vi "Convert Error Cluster to Table.vi"(11 "Error Codes":cluster{i32, string}[](array[cluster])) -> (2 "Code":i32[](array[numeric]), 3 "String":string[](array[string]))   [LabVIEW 2019, in "Ghost Bus Addon System Explorer.lvlib"] (continued)
of the remote endpoint does not match the data type of the local endpoint. The data types of the endpoints must match."}, {-314240, "LabVIEW: (Hex 0xFFFB3480) The stream detected an unrecoverable loss of data.  Contact National Instruments for support."}, {-314235, "LabVIEW: (Hex 0xFFFB3485) The remote endpoint was restarted because the computer that hosts the endpoint crashed, was rebooted, or experienced a hang."}, {-314230, "LabVIEW: (Hex 0xFFFB348A) LabVIEW could not create the local endpoint because the computer that hosts the endpoint ran out of memory."}, {-314227, "LabVIEW: (Hex 0xFFFB348D) The URL you specified with the reader url or writer url terminal does not include the name of the remote endpoint. You must specify a valid endpoint URL in one of these terminals to connect two endpoints together."}, {-314226, "LabVIEW: (Hex 0xFFFB348E) Incompatible format."}, {-314220, "LabVIEW: (Hex 0xFFFB3494) The remote endpoint has been destroyed."}, {-314215, "LabVIEW: (Hex 0xFFFB3499) You cannot read or write a number of elements that is larger than the size of the endpoint buffer."}, {-314202, "LabVIEW: (Hex 0xFFFB34A6) You cannot flush a network stream from the reader endpoint. Call the Flush Stream function from the writer endpoint only."}, {-314201, "LabVIEW: (Hex 0xFFFB34A7) The local endpoint lost connection and reconnected with the remote endpoint, but some data was lost."}, {-314109, "LabVIEW: (Hex 0xFFFB3503) The name of one endpoint cannot be the partial name of another endpoint within the same application.  Change the name of this endpoint so that it does not overlap with an existing name, or destroy the other endpoint before creating this endpoint."}, {-314108, "LabVIEW: (Hex 0xFFFB3504) The name of one endpoint cannot be the partial name of another endpoint within the same application.  Change the name of this endpoint so that it does not overlap with an existing name, or destroy the other endpoint before creating this endpoint."}, {-314107, "LabVIEW: (Hex 0xFFFB3505) The local endpoint is already connected to another endpoint. Each endpoint can connect to only one other endpoint at a time."}, {-314106, "LabVIEW: (Hex 0xFFFB3506) The local endpoint is not connected to a remote endpoint. Specify the URL of a remote endpoint in the writer url terminal of the Create Network Stream Reader Endpoint function or the reader url terminal of the Create Network Stream Writer Endpoint function to prompt a connection between two endpoints."}, {-314105, "LabVIEW: (Hex 0xFFFB3507) You can call the Write Single Element to Stream and Write Multiple Elements to Stream functions from the writer endpoint only."}, {-314104, "LabVIEW: (Hex 0xFFFB3508) You can call the Read Single Element from Stream and Read Multiple Elements from Stream functions from the reader endpoint only."}, {-314103, "LabVIEW: (Hex 0xFFFB3509) You did not specify an endpoint name. Specify a valid name or endpoint URL with the reader name terminal of the Create Network Stream Reader Endpoint function or the writer name terminal of the Create Network Stream Writer Endpoint function."}, {-314102, "LabVIEW: (Hex 0xFFFB350A) The buffer size of the endpoint must be greater than zero elements."}, {-314101, "LabVIEW: (Hex 0xFFFB350B) An endpoint with the same name already exists."}, {-314100, "LabVIEW: (Hex 0xFFFB350C) The specified endpoint does not exist."}, {-314054, "LabVIEW: (Hex 0xFFFB353A) The Network Streams Engine cannot be uninitialized."}, {-314053, "LabVIEW: (Hex 0xFFFB353B) The Network Streams Engine failed to initialize."}, {-314052, "LabVIEW: (Hex 0xFFFB353C) The Network Streams Engine is not initialized."}, {-314051, "LabVIEW: (Hex 0xFFFB353D) The Network Streams Engine was already initialized."}, {-314050, "LabVIEW: (Hex 0xFFFB353E) The Network Streams Engine does not exist."}, {-314009, "LabVIEW: (Hex 0xFFFB3567) The value wired to the Wait Condition input is invalid. Refer to the LabVIEW Help for valid values."}, {-314008, "LabVIEW: (Hex 0xFFFB3568) The value wired to the Element Allocation Mode input is invalid. Refer to the LabVIEW Help for valid values."}, {-314007, "LabVIEW: (Hex 0xFFFB3569) You cannot read multiple array elements of different dimensions. You can read multiple array elements of the same dimension only."}, {-314006, "LabVIEW: (Hex 0xFFFB356A) You cannot specify a relative URL with the reader url and writer url terminals. You must use an absolute URL instead. For example,  if you are connecting to an endpoint with the name Endpoint1 on a computer with the IP address 10.0.0.62, use the URL //10.0.0.62/stream1."}, {-314005, "LabVIEW: (Hex 0xFFFB356B) The ni_nwstreams library contains invalid parameters."}, {-314004, "LabVIEW: (Hex 0xFFFB356C) LabVIEW could not create the endpoint within the timeout period. Ensure that you specify the URL of a remote endpoint with the reader url terminal of the Create Network Stream Writer Endpoint function or the writer url terminal of the Create Network Stream Reader Endpoint function."}, {-314003, "LabVIEW: (Hex 0xFFFB356D) LabVIEW could not create a network stream. You must specify the URL of a remote endpoint with either the reader url terminal of the Create Network Stream Writer Endpoint function or the writer url terminal of the Create Network Stream Reader Endpoint function."}, {-314002, "LabVIEW: (Hex 0xFFFB356E) You cannot call this property from the reader endpoint. You can call this property from the writer endpoint only."}, {-314001, "LabVIEW: (Hex 0xFFFB356F) You cannot call this property from the writer endpoint. You can call this property from the reader endpoint only."}, {-314000, "LabVIEW: (Hex 0xFFFB3570) LabVIEW cannot load the ni_nwstreams library. If you are using a desktop computer, you might need to repair your LabVIEW installation or reinstall LabVIEW or the LabVIEW Run-Time Engine. If you are using an RT target, verify that you installed the network streams feature with Measurement and Automation Explorer (MAX)."}, {-311119, "LabVIEW: (Hex 0xFFFB40B1) Failed to connect to the MAX database (MXS) when undeploying the EPICS Client I/O server."}, {-311118, "LabVIEW: (Hex 0xFFFB40B2) Failed to connect to the MAX database (MXS) when deploying the EPICS Client I/O server."}, {-311117, "LabVIEW: (Hex 0xFFFB40B3) Failed to connect to the MAX database (MXS) when creating the EPICS Client I/O server."}, {-311116, "LabVIEW: (Hex 0xFFFB40B4) The specified access type is invalid for the EPICS Client I/O server."}, {-311115, "LabVIEW: (Hex 0xFFFB40B5) The specified data type is invalid for the EPICS Client I/O server."}, {-311114, "LabVIEW: (Hex 0xFFFB40B6) Unable to find the specified field name on the EPICS Client I/O server."}, {-311113, "LabVIEW: (Hex 0xFFFB40B7) Unable to find the specified record name on the EPICS Client I/O server."}, {-311111, "LabVIEW: (Hex 0xFFFB40B9) Failed to locate a network interface. Make sure you have properly configured a network interface. Then deploy the EPICS Server I/O server again."}, {-311110, "LabVIEW: (Hex 0xFFFB40BA) Failed to load EPICS Base libraries. Make sure you have properly installed EPICS Base libraries."}, {-311109, "LabVIEW: (Hex 0xFFFB40BB) The specified process variable (PV) name includes an invalid character. The valid character set for a PV name is: a-z, A-Z, 0-9, _, -, :, ., [, ], <, >, ;."}, {-311108, "LabVIEW: (Hex 0xFFFB40BC) Unable to locate the process variable (PV)."}, {-311107, "LabVIEW: (Hex 0xFFFB40BD) Failed to connect to the MAX database (MXS) when removing an empty process or folder."}, {-311106, "LabVIEW: (Hex 0xFFFB40BE) Failed to connect to the MAX database (MXS) when undeploying the EPICS Server I/O server."}, {-311105, "LabVIEW: (Hex 0xFFFB40BF) Failed to connect to the MAX database (MXS) when deploying the EPICS Server I/O server."}, {-311104, "LabVIEW: (Hex 0xFFFB40C0) Failed to connect to the MAX database (MXS) when creating a process or folder."}, {-311103, "LabVIEW: (Hex 0xFFFB40C1) Failed to connect to the MAX database (MXS) when creating the EPICS Server I/O server."}, {-311102, "LabVIEW: (Hex 0xFFFB40C2) The specified process variable (PV) name conflicts with an existing PV name."}, {-311101, "LabVIEW: (Hex 0xFFFB40C3) The variable path must be a valid absolute URL or a machine-relative URL."}, {-311100, "LabVIEW: (Hex 0xFFFB40C4) Not a URL or an invalid URL. The EPICS Client URL or EPICS Server URL must be an absolute URL or a machine-relative URL."}, {-311071, "LabVIEW: (Hex 0xFFFB40E1) Unable to run the built application on the target. A user must log into a Windows session on the target."}, {-311070, "LabVIEW: (Hex 0xFFFB40E2) Unable to run the built application on the target. The target returns an unexpected error."}, {-311052, "LabVIEW: (Hex 0xFFFB40F4) Cannot commit all files."}, {-311051, "LabVIEW: (Hex 0xFFFB40F5) FBWF returned an unknown error."}, {-311050, "LabVIEW: (Hex 0xFFFB40F6) Cannot find the FBWF cache entry."}, {-311049, "LabVIEW: (Hex 0xFFFB40F7) The system does not have enough memory to list all the FBWF cache entries."}, {-311048, "LabVIEW: (Hex 0xFFFB40F8) The file path to remove does not exist in the exclusion list for the next session."}, {-311047, "LabVIEW: (Hex 0xFFFB40F9) The file to restore does not exist in the FBWF cache."}, {-311046, "LabVIEW: (Hex 0xFFFB40FA) Cannot restore a read-only file."}, {-311045, "LabVIEW: (Hex 0xFFFB40FB) Cannot restore the file, because the file is in the exclusion path, renamed, or does not exist on the physical media."}, {-311044, "LabVIEW: (Hex 0xFFFB40FC) Cannot commit changes, because the file is write-protected. For example, the file is in the CD-ROM."}, {-311043, "LabVIEW: (Hex 0xFFFB40FD) Cannot commit changes, because the file is in the exclusion path, renamed, or does not exist on the physical media."}, {-311042, "LabVIEW: (Hex 0xFFFB40FE) The file is not valid or not in the FBWF cache."}, {-311041, "LabVIEW: (Hex 0xFFFB40FF) The volume name is not valid or the volume is not protected by FBWF."}, {-311040, "LabVIEW: (Hex 0xFFFB4100) FBWF is currently disabled, not enabled for the next session, or the volume is not protected by FBWF."}, {-311026, "LabVIEW: (Hex 0xFFFB410E) Failed to set a checkpoint level on the EWF protected volume."}, {-311025, "LabVIEW: (Hex 0xFFFB410F) Failed to free the memory that the EWF uses."}, {-311024, "LabVIEW: (Hex 0xFFFB4110) Failed to get the configuration information of the EWF protected volume."}, {-311023, "LabVIEW: (Hex 0xFFFB4111) Failed to get the configuration information of the EWF storage volume."}, {-311022, "LabVIEW: (Hex 0xFFFB4112) Failed to open the EWF overlay storage volume."}, {-311021, "LabVIEW: (Hex 0xFFFB4113) Failed to restore an EWF protected volume."}, {-311020, "LabVIEW: (Hex 0xFFFB4114) Failed to create a new checkpoint on the EWF protected volume."}, {-311019, "LabVIEW: (Hex 0xFFFB4115) Failed to disable HORM on the EWF protected volume."}, {-311018, "LabVIEW: (Hex 0xFFFB4116) Failed to enable HORM on the EWF protected volume."}, {-311017, "LabVIEW: (Hex 0xFFFB4117) Failed to get the list of EWF protected volumes."}, {-311016, "LabVIEW: (Hex 0xFFFB4118) Failed to clear the EWF command on the EWF protected volume."}, {-311015, "LabVIEW: (Hex 0xFFFB4119) Failed to live commit changes and disable EWF on the EWF protected volume."}, {-311014, "LabVIEW: (Hex 0xFFFB411A) Failed to commit changes to the EWF protected volume."}, {-311013, "LabVIEW: (Hex 0xFFFB411B) Failed to disable EWF on the volume."}, {-311012, "LabVIEW: (Hex 0xFFFB411C) Failed to enable EWF on the volume."}, {-311011, "LabVIEW: (Hex 0xFFFB411D) Failed to close the EWF protected volume handle or the EWF storage volume handle."}, {-311010, "LabVIEW: (Hex 0xFFFB411E) Failed to open the EWF protected volume."}, {-311001, "LabVIEW: (Hex 0xFFFB4127) Failed to get the Write Filters VIs library function."}, {-311000, "LabVIEW: (Hex 0xFFFB4128) Failed to load the Write Filters VIs library."}, {-124201, "LabVIEW: (Hex 0xFFFE1AD7) An unknown internal error has occurred."}, {-124110, "LabVIEW: (Hex 0xFFFE1B32) The server does not recognize the specified request."}, {-124109, "LabVIEW: (Hex 0xFFFE1B33) The user specified a resource that exists on a different server."}, {-124108, "LabVIEW: (Hex 0xFFFE1B34) Cannot close session because requests are still open."}, {-124107, "LabVIEW: (Hex 0xFFFE1B35) The user specified an invalid DAV resource."}, {-124106, "LabVIEW: (Hex 0xFFFE1B36) The operation cannot be performed because the resource is locked."}, {-124105, "LabVIEW: (Hex 0xFFFE1B37) The specified request is missing a precondition, specified by the server (perhaps an HTTP header)."}, {-124104, "LabVIEW: (Hex 0xFFFE1B38) The server does not support the request body type."}, {-124103, "LabVIEW: (Hex 0xFFFE1B39) The requested resource does not support the specified DAV method. Ensure there is a WebDAV server installed on the host and enabled on the specified port. When communicating with LabVIEW Real-Time targets, specify /files as the URI prefix."}, {-124102, "LabVIEW: (Hex 0xFFFE1B3A) The request could not be completed due to a conflict with the current state of the resource."}, {-124101, "LabVIEW: (Hex 0xFFFE1B3B) The property change could not be made because another property change also failed."}, {-124100, "LabVIEW: (Hex 0xFFFE1B3C) The requested resource was not found."}, {-124004, "LabVIEW: (Hex 0xFFFE1B9C) Cannot accept new DAV requests because the DAV engine is shutting down."}, {-124003, "LabVIEW: (Hex 0xFFFE1B9D) A request is already pending."}, {-124002, "LabVIEW: (Hex 0xFFFE1B9E) The specified request handle is invalid."}, {-124001, "LabVIEW: (Hex 0xFFFE1B9F) The specified session handle is invalid."}, {-120000, "LabVIEW: (Hex 0xFFFE2B40) SignalExpress is required to open this Express VI.  Install SignalExpress or visit www.ni.com/signalexpress to download an evaluation version."}, {-90165, "LabVIEW: (Hex 0xFFFE9FCB) A command occurred that is only supported within a loop, such as a For Loop or a While Loop."}, {-90164, "LabVIEW: (Hex 0xFFFE9FCC) An unidentified error occurred in the parser."}, {-90163, "LabVIEW: (Hex 0xFFFE9FCD) The parser aborted recognition of a token."}, {-90162, "LabVIEW: (Hex 0xFFFE9FCE) A recognition error occurred while generating a stream of tokens."}, {-90161, "LabVIEW: (Hex 0xFFFE9FCF) An I/O error occurred while generating a stream of tokens."}, {-90160, "LabVIEW: (Hex 0xFFFE9FD0) An unidentified error occurred while generating a stream of tokens."}, {-90159, "LabVIEW: (Hex 0xFFFE9FD1) A semantic error occurred while parsing."}, {-90158, "LabVIEW: (Hex 0xFFFE9FD2) LabVIEW found an unexpected character while parsing."}, {-90157, "LabVIEW: (Hex 0xFFFE9FD3) LabVIEW found an unexpected token while parsing."}, {-90156, "LabVIEW: (Hex 0xFFFE9FD4) LabVIEW found a mismatched token while parsing."}, {-90155, "LabVIEW: (Hex 0xFFFE9FD5) LabVIEW found a mismatched character while parsing."}, {-90154, "LabVIEW: (Hex 0xFFFE9FD6) An unidentified error occurred while attempting to recognize a character or token."}, {-90153, "LabVIEW: (Hex 0xFFFE9FD7) An I/O error occurred while generating a stream of characters."}, {-90152, "LabVIEW: (Hex 0xFFFE9FD8) An unidentified error occurred while generating a stream of characters."}, {-90151, "LabVIEW: (Hex 0xFFFE9FD9) A parser error occurred."}, {-90149, "LabVIEW: (Hex 0xFFFE9FDB) The MathScript RT Module is not installed on this computer, has expired, or is licensed invalidly. Install or activate the LabVIEW MathScript RT Module on this computer to continue using this product. Visit the National Instruments Web site at ni.com to purchase these products. If you have already purchased this product, select <b>Help>>Activate LabVIEW Components</b> to activate this product."}, {-90148, "LabVIEW: (Hex 0xFFFE9FDC) The MathScript RT Module requires the LabVIEW Full or Professional Development Systems, LabVIEW Debug Deployment System, or LabVIEW Student Edition to run correctly.  Visit the National Instruments Web site at ni.com to purchase these products. If you have already purchased one of these products, select <b>Help>>Activate LabVIEW Components</b> to activate the product."}, {-90147, "LabVIEW: (Hex 0xFFFE9FDD) The MathScript parser DLL is missing or corrupt. You might need to reinstall LabVIEW to correct this issue."}, {-90146, "LabVIEW: (Hex 0xFFFE9FDE) Invalid output data type. The output terminal to the MathScript Node breaks if you attempt to pass a structure with a field that is a plot object."}, {-90145, "LabVIEW: (Hex 0xFFFE9FDF) Invalid output data type. The output terminal to the MathScript Node breaks if you attempt to pass a structure with a field that is not known until run time."}, {-90144, "LabVIEW: (Hex 0xFFFE9FE0) Invalid output data type. The output terminal to the MathScript Node breaks if you attempt to pass a dynamic structure."}, {-90143, "LabVIEW: (Hex 0xFFFE9FE1) Invalid output data type. You cannot pass a cell array of any data type other than string out of the MathScript Node."}, {-90131, "LabVIEW: (Hex 0xFFFE9FED) This variable depends upon an input to the function that is unwired."}, {-90130, "LabVIEW: (Hex 0xFFFE9FEE) This function is not supported on the current hardware target."}, {-90129, "LabVIEW: (Hex 0xFFFE9FEF) LabVIEW cannot coerce the output to the desired data type."}, {-90128, "LabVIEW: (Hex 0xFFFE9FF0) You cannot use the : operator as a parameter to a function.  You can use : only in a variable indexing operation."}, {-90127, "LabVIEW: (Hex 0xFFFE9FF1) The function as written will be ignored in the LabVIEW Run-Time Engine."}, {-90126, "LabVIEW: (Hex 0xFFFE9FF2) All columns of a matrix must have the same number of rows."}, {-90125, "LabVIEW: (Hex 0xFFFE9FF3) The LabVIEW MathScript function is not available on this platform."}, {-90124, "LabVIEW: (Hex 0xFFFE9FF4) Arguments to the global or persistent functions must be string literals."}, {-90123, "LabVIEW: (Hex 0xFFFE9FF5) The global and persistent keywords are reserved for the global and persistent built-in functions, and you cannot use those words to name a function or a script."}, {-90122, "LabVIEW: (Hex 0xFFFE9FF6) The global and persistent keywords are reserved for the global and persistent built-in functions, and you cannot use those words as variables."}, {-90121, "LabVIEW: (Hex 0xFFFE9FF7) LabVIEW did not locate the requested function in the .m file."}, {-90120, "LabVIEW: (Hex 0xFFFE9FF8) The function you specified as an argument contains an incorrect syntax. Make sure that the function has the correct data types and the correct number of inputs and outputs described by the help."}, {-90119, "LabVIEW: (Hex 0xFFFE9FF9) The <b>times</b> input of the ode function must contain at least two elements, and these elements must be strictly monotonic."}, {-90118, "LabVIEW: (Hex 0xFFFE9FFA) A return command occurred that is supported only within a user-defined function or script."}, {-90117, "LabVIEW: (Hex 0xFFFE9FFB) A continue command occurred that is supported only within a loop, such as a For Loop or a While Loop."}, {-90116, "LabVIEW: (Hex 0xFFFE9FFC) A break command occurred that is supported only within a loop, such as a For Loop or a While Loop."}, {-90115, "LabVIEW: (Hex 0xFFFE9FFD) The specified attribute is read-only."}, {-90114, "LabVIEW: (Hex 0xFFFE9FFE) The specified attribute name or attribute value is invalid."}, {-90113, "LabVIEW: (Hex 0xFFFE9FFF) The specified object no longer exists or is corrupt."}, {-90112, "LabVIEW: (Hex 0xFFFEA000) An internal error occurred while processing this MathScript. Contact National Instruments with the MathScript you used."}, {-90111, "LabVIEW: (Hex 0xFFFEA001) Cannot find the function you specified as an argument. Make sure the function is saved in the LabVIEW Data directory or a directory in the MathScript search path list."}, {-90110, "LabVIEW: (Hex 0xFFFEA002) This function can be called only in the <b>LabVIEW MathScript Window</b>."}, {-90109, "LabVIEW: (Hex 0xFFFEA003) The operating system reported a problem while trying to unload the shared library."}, {-90108, "LabVIEW: (Hex 0xFFFEA004) You cannot call a function with the requested type of input."}, {-90107, "LabVIEW: (Hex 0xFFFEA005) The function you requested does not exist in the shared library."}, {-90106, "LabVIEW: (Hex 0xFFFEA006) You cannot call shared library functions with numeric pointer return types from MathScript."}, {-90105, "LabVIEW: (Hex 0xFFFEA007) The shared library function expects a value but was called with a matrix."}, {-90104, "LabVIEW: (Hex 0xFFFEA008) LabVIEW could not parse the header file correctly."}, {-90103, "LabVIEW: (Hex 0xFFFEA009) The operating system could not load the shared library because a problem was reported."}, {-90102, "LabVIEW: (Hex 0xFFFEA00A) LabVIEW could not call the function from the shared library."}, {-90101, "LabVIEW: (Hex 0xFFFEA00B) LabVIEW could not return a string from the shared library call."}, {-90100, "LabVIEW: (Hex 0xFFFEA00C) LabVIEW could not find the specified function in the header file."}, {-90099, "LabVIEW: (Hex 0xFFFEA00D) The shared library you requested is not loaded."}, {-90098, "LabVIEW: (Hex 0xFFFEA00E) A shared library with the specified name or alias already is loaded."}, {-90097, "LabVIEW: (Hex 0xFFFEA00F) LabVIEW could not find the header file in the search path."}, {-90096, "LabVIEW: (Hex 0xFFFEA010) LabVIEW could not find the shared library in the search path."}, {-90095, "LabVIEW: (Hex 0xFFFEA011) The input parameters must be integers less than bitmax."}, {-90094, "LabVIEW: (Hex 0xFFFEA012) This is a custom error message generated in the script."}, {-90093, "LabVIEW: (Hex 0xFFFEA013) The LabVIEW Run-Time Engine does not support this function."}, {-90092, "LabVIEW: (Hex 0xFFFEA014) The end keyword is valid only as part of a matrix indexing operation. This error can occur when you attempt to use end without an associated variable."}, {-90091, "LabVIEW: (Hex 0xFFFEA015) The specified range is too large."}, {-90090, "LabVIEW: (Hex 0xFFFEA016) The user function signature contains an incorrect number of outputs. It must contain one output."}, {-90089, "LabVIEW: (Hex 0xFFFEA017) The user function signature contains an incorrect number of inputs. It must contain two inputs."}, {-90088, "LabVIEW: (Hex 0xFFFEA018) A switch statement supports only scalar elements and strings."}, {-90087, "LabVIEW: (Hex 0xFFFEA019) The given function name does not correspond to a known function."}, {-90086, "LabVIEW: (Hex 0xFFFEA01A) LabVIEW cannot compile the current MathScript. Contact National Instruments with the MathScript you used."}, {-90084, "LabVIEW: (Hex 0xFFFEA01C) You tried to pass an input of an unexpected data type to the .m file or the .m file output is of an unexpected data type. The two inputs and the output must all be double vectors."}, {-90083, "LabVIEW: (Hex 0xFFFEA01D) MathScript cannot open the user-defined function. This could be due to a missing .m file or an incorrect search path."}, {-90082, "LabVIEW: (Hex 0xFFFEA01E) The fields of the structure you want to reorder do not match the fields of the model structure."}, {-90081, "LabVIEW: (Hex 0xFFFEA01F) The permutation array must have the same length as the number of fields in the structure you want to reorder."}, {-90080, "LabVIEW: (Hex 0xFFFEA020) Cannot find the field you specified within the structure."}, {-90079, "LabVIEW: (Hex 0xFFFEA021) You specified an invalid format specifier."}, {-90078, "LabVIEW: (Hex 0xFFFEA022) The sizes of the input matrices are incompatible."}, {-90077, "LabVIEW: (Hex 0xFFFEA023) Invalid input data type. You cannot pass a structure with an invalid input data type into the MathScript Node."}, {-90076, "LabVIEW: (Hex 0xFFFEA024) You cannot use the \".\" operator to dereference data that is not a structure."}, {-90075, "LabVIEW: (Hex 0xFFFEA025) Field names must be strings."}, {-90072, "LabVIEW: (Hex 0xFFFEA028) You specified an empty matrix."}, {-90071, "LabVIEW: (Hex 0xFFFEA029) Field names must begin with an alphabetic character. Field names can contain only alphanumeric characters and underscores."}, {-90070, "LabVIEW: (Hex 0xFFFEA02A) The lengths of the two input vectors are not compatible."}, {-90069, "LabVIEW: (Hex 0xFFFEA02B) MathScript can only dereference individual structure elements. You must index the structure array before you can dereference."}, {-90068, "LabVIEW: (Hex 0xFFFEA02C) You cannot dereference a field that does not exist within the structure."}, {-90067, "LabVIEW: (Hex 0xFFFEA02D) The elements of the input vector must be in increasing order."}, {-90066, "LabVIEW: (Hex 0xFFFEA02E) NI-DAQmx is not installed or might be corrupted. Install or repair the NI-DAQmx software."}, {-90065, "LabVIEW: (Hex 0xFFFEA02F) The values of the input vectors are not compatible."}, {-90064, "LabVIEW: (Hex 0xFFFEA030) All elements of the input vector must be positive."}, {-90063, "LabVIEW: (Hex 0xFFFEA031) All real elements of the input vector must be greater than or equal to 0."}, {-90062, "LabVIEW: (Hex 0xFFFEA032) All input elements must be in the interval [-1, 1]."}, {-90061, "LabVIEW: (Hex 0xFFFEA033) You specified an empty vector."}, {-90060, "LabVIEW: (Hex 0xFFFEA034) This function requires the LabVIEW Real-Time Execution Trace Toolkit 2.0 or later, but the toolkit is either not installed or not licensed properly."}, {-90059, "LabVIEW: (Hex 0xFFFEA035) The input parameter must be a vector."}, {-90058, "LabVIEW: (Hex 0xFFFEA036) The variable is defined within the script, but the code that defines the variable did not execute."}, {-90057, "LabVIEW: (Hex 0xFFFEA037) The input scalar must be in the interval [0, 1]."}, {-90056, "LabVIEW: (Hex 0xFFFEA038) The input scalar cannot be 0."}, {-90055, "LabVIEW: (Hex 0xFFFEA039) The input scalar must be positive."}, {-90054, "LabVIEW: (Hex 0xFFFEA03A) The input scalar must be greater than or equal to 0."}, {-90053, "LabVIEW: (Hex 0xFFFEA03B) You can specify only one or two index arguments, such as a(1, 2)."}, {-90052, "LabVIEW: (Hex 0xFFFEA03C) You specified an invalid number of output parameters for this function."}, {-90051, "LabVIEW: (Hex 0xFFFEA03D) You specified an invalid number of input parameters for this function."}, {-90050, "LabVIEW: (Hex 0xFFFEA03E) You cannot specify a step size of zero for a range."}, {-90049, "LabVIEW: (Hex 0xFFFEA03F) The input parameters must be real, positive numbers."}, {-90048, "LabVIEW: (Hex 0xFFFEA040) You must call the timerstart function before calling the timerstop function."}, {-90047, "LabVIEW: (Hex 0xFFFEA041) You must use a square matrix."}, {-90046, "LabVIEW: (Hex 0xFFFEA042) The input parameters are not in the required format."}, {-90045, "LabVIEW: (Hex 0xFFFEA043) The base of the number conversion must be an integer between 2 and 36."}, {-90044, "LabVIEW: (Hex 0xFFFEA044) You must operate on the first or second dimension."}, {-90043, "LabVIEW: (Hex 0xFFFEA045) The matrix sizes are not valid."}, {-90042, "LabVIEW: (Hex 0xFFFEA046) The data types you specified are incompatible. This error can occur when you build a matrix with elements of different data types."}, {-90041, "LabVIEW: (Hex 0xFFFEA047) All rows of a matrix must have the same number of columns."}, {-90040, "LabVIEW: (Hex 0xFFFEA048) The sizes of the inputs are incompatible. Verify that x, y, and z have the same size or that the length of x and y equal the number of columns and rows of z."}, {-90039, "LabVIEW: (Hex 0xFFFEA049) You cannot convert a Boolean to a character. This error can occur when you replace a character matrix element with a Boolean or when you explicitly convert a Boolean to a character."}, {-90038, "LabVIEW: (Hex 0xFFFEA04A) You cannot convert a uint64 number to a Boolean.  This error can occur when you replace a Boolean matrix element with a uint64 element or when you explicitly convert a uint64 number to a Boolean."}, {-90037, "LabVIEW: (Hex 0xFFFEA04B) You cannot convert an int64 number to a Boolean.  This error can occur when you replace a Boolean matrix element with an int64 element or when you explicitly convert an int64 number to a Boolean."}, {-90036, "LabVIEW: (Hex 0xFFFEA04C) You cannot convert a character to a Boolean.  This error can occur when you replace a Boolean matrix element with a character or when you explicitly convert a character to a Boolean."}, {-90035, "LabVIEW: (Hex 0xFFFEA04D) You cannot convert a complex number to a Boolean.  This error can occur when you replace a Boolean matrix element with a complex element or when you explicitly convert a complex number to a Boolean."}, {-90034, "LabVIEW: (Hex 0xFFFEA04E) The number of rows and columns that the indexes specify must equal the number of rows and columns of values you want to set."}, {-90033, "LabVIEW: (Hex 0xFFFEA04F) You cannot use an empty matrix to delete a single element in a 2D matrix."}, {-90032, "LabVIEW: (Hex 0xFFFEA050) The indexes are out of bounds for the variable you specified."}, {-90031, "LabVIEW: (Hex 0xFFFEA051) The given name does not correspond to a known function, variable, or symbol."}, {-90030, "LabVIEW: (Hex 0xFFFEA052) You cannot resize a 2D matrix by indexing the matrix with a linear index that is out of the bounds of the matrix."}, {-90029, "LabVIEW: (Hex 0xFFFEA053) You cannot replace elements of a matrix with elements of non-matrix data types, such as plot objects and state-space, transfer function, and zero-pole-gain models."}, {-90028, "LabVIEW: (Hex 0xFFFEA054) The number of indexes must match the number of values you want to assign to a matrix."}, {-90027, "LabVIEW: (Hex 0xFFFEA055) You cannot index a variable of a non-matrix data type, such as a plot object or a state-space, transfer function, or zero-pole-gain model."}, {-90026, "LabVIEW: (Hex 0xFFFEA056) The indexes for a matrix indexing operation must be real, positive integers."}, {-90025, "LabVIEW: (Hex 0xFFFEA057) The file identifier you specified is invalid.  Make sure LabVIEW opened the file successfully."}, {-90024, "LabVIEW: (Hex 0xFFFEA058) LabVIEW does not understand the optional parameter you passed to this function. Verify that you spelled the parameter correctly and that the option is valid for this function."}, {-90023, "LabVIEW: (Hex 0xFFFEA059) The data type of the input parameters is not valid for this operation."}, {-90022, "LabVIEW: (Hex 0xFFFEA05A) LabVIEW does not understand the parameters you passed to this function."}, {-90021, "LabVIEW: (Hex 0xFFFEA05B) This function does not operate on matrices of 3 or more dimensions."}, {-90020, "LabVIEW: (Hex 0xFFFEA05C) LabVIEW cannot display the content of a plug-in data type on RT."}, {-90019, "LabVIEW: (Hex 0xFFFEA05D) This operation requires at least one parameter to be a scalar."}, {-90018, "LabVIEW: (Hex 0xFFFEA05E) The input parameters for this function must be real."}, {-90017, "LabVIEW: (Hex 0xFFFEA05F) The bit you want to set is outside the range of the current floating-point representation."}, {-90016, "LabVIEW: (Hex 0xFFFEA060) The bit you want to get is outside the range of the current floating-point representation."}, {-90015, "LabVIEW: (Hex 0xFFFEA061) If you perform a bitwise complement and treat the result as an N-bit number, the original number cannot be greater than 2^N."}, {-90014, "LabVIEW: (Hex 0xFFFEA062) The input parameters must be nonnegative integers less than bitmax."}, {-90013, "LabVIEW: (Hex 0xFFFEA063) Elements of the input matrices must be nonnegative integers of the same data type."}, {-90012, "LabVIEW: (Hex 0xFFFEA064) You cannot use this function in a MathScript Node that is not on an RT target."}, {-90011, "LabVIEW: (Hex 0xFFFEA065) The sizes of the input matrices are incompatible.  Verify that the matrices have the same size or that one is a scalar."}, {-90010, "LabVIEW: (Hex 0xFFFEA066) The inputs to this function must be scalar."}, {-90009, "LabVIEW: (Hex 0xFFFEA067) The operator you want to use is not defined. If the operator is correct, contact National Instruments."}, {-90008, "LabVIEW: (Hex 0xFFFEA068) This function is not defined to operate on complex data. This error can occur when you perform a logical operation with invalid data types."}, {-90007, "LabVIEW: (Hex 0xFFFEA069) This function is not defined to operate on Boolean, character, or single-precision data. This error can occur when you perform a bitwise operation with invalid data types."}, {-90006, "LabVIEW: (Hex 0xFFFEA06A) This function is defined to operate only on letters of the ISO-8859-1 character set"}, {-90005, "LabVIEW: (Hex 0xFFFEA06B) An output variable of the user-defined function is undefined. The output variable might be defined in the body of a case structure or a loop in the .m file that does not execute at run time."}, {-90004, "LabVIEW: (Hex 0xFFFEA06C) This function is not defined for non-numeric data types."}, {-90003, "LabVIEW: (Hex 0xFFFEA06D) This function is not defined for the number of parameters you supplied."}, {-90002, "LabVIEW: (Hex 0xFFFEA06E) You must wire a valid data type to this input or delete the input."}, {-90001, "LabVIEW: (Hex 0xFFFEA06F) A problem occurred in a subVI call."}, {-68027, "LabVIEW: (Hex 0xFFFEF645) The TDMS Defragment, TDMS Convert Format, and TDMS Delete Data functions cannot process a file that has a TDMS segment containing data from multiple groups with interleaved channels. Data can be read from the file using the TDMS Read function."}, {-68026, "LabVIEW: (Hex 0xFFFEF646) Failed to delete data from the .tdms file, because <b>channel names</b> contains digital data."}, {-68025, "LabVIEW: (Hex 0xFFFEF647) Failed to delete the index file after writing data to the TDMS file. National Instruments recommends that you delete the index file manually."}, {-68024, "LabVIEW: (Hex 0xFFFEF648) The TDM Streaming VIs and Functions do not support extended-precision floating-point numbers on Linux, OS X, and VxWorks."}, {-68023, "LabVIEW: (Hex 0xFFFEF649) The value is out of range. Set the block size between 1KB and 1GB."}, {-68022, "LabVIEW: (Hex 0xFFFEF64A) Failed to append data to a TDMS in-memory file because the TDMS In Memory Read Bytes function has been called."}, {-68021, "LabVIEW: (Hex 0xFFFEF64B) Failed to reset the memory block size because data has written to the in-memory TDMS file reference. Reset the block size before writing data."}, {-68020, "LabVIEW: (Hex 0xFFFEF64C) This file reference is an in-memory TDMS file reference. Use TDMS functions that support the in-memory TDMS file reference."}, {-68019, "LabVIEW: (Hex 0xFFFEF64D) This function or property is supported by the in-memory TDMS file reference only. Use the TDMS In Memory Open function to open the file reference."}, {-68018, "LabVIEW: (Hex 0xFFFEF64E) Failed to update the .tdms file. This file might be incomplete due to an application crash during the logging process. You can still read the existing data from this file, but you cannot append new data to this file. Consider creating a new .tdms file for your application."}, {-68017, "LabVIEW: (Hex 0xFFFEF64F) The hierarchy of certain channels or groups in the file is not supported by the current version of LabVIEW. Upgrade LabVIEW to the latest version to fix this error. Contact National Instruments if this error persists."}, {-68016, "LabVIEW: (Hex 0xFFFEF650) The data in certain channels or groups of the file is not supported. LabVIEW skips these channels or groups when listing content of the file. Upgrade LabVIEW to the latest version to fix this error. Contact National Instruments if this error persists."}, {-68015, "LabVIEW: (Hex 0xFFFEF651) This channel contains multi-dimension data that is not recognized by the current version of LabVIEW. Upgrade LabVIEW to the latest version to fix this error. Contact National Instruments if this error persists."}, {-68014, "LabVIEW: (Hex 0xFFFEF652) Failed to append data to the specified channel because the dimension of the new data does not match that of the existing data."}, {-68013, "LabVIEW: (Hex 0xFFFEF653) Failed to access the specified channel because this channel is protected by LabVIEW. You cannot rename the group that contains the protected channel because renaming a group affects all channel names under that group. If you are creating a new channel or renaming an existing channel, use another channel name."}, {-68010, "LabVIEW: (Hex 0xFFFEF656) File is still in use. Close all other references to this file before truncating the file."}, {-68009, "LabVIEW: (Hex 0xFFFEF657) TDMS asynchronous mode is not initialized properly. Make sure the <b>enable asynchronous?</b> input of the TDMS Advanced Open function is TRUE. If you are writing data to a file, also make sure the TDMS Configure Asynchronous Writes (Data Ref) function exists. If you are reading data from a file, also make sure the TDMS Configure Asynchronous Reads (Data Ref) function exists."}, {-68008, "LabVIEW: (Hex 0xFFFEF658) The <b>data type</b> input of the TDMS Configure Asynchronous Writes function is not wired. If the <b>pre-allocate?</b> input of this function is TRUE, you must wire a supported <b>data type</b> to this function. LabVIEW uses the data type information to determine the size of each pre-allocated buffer. The <b>data type</b> input accepts integers, floating-point numbers, Booleans, and timestamps."}, {-68007, "LabVIEW: (Hex 0xFFFEF659) This channel or property value contains a data type that is not recognized by this version of LabVIEW."}, {-68006, "LabVIEW: (Hex 0xFFFEF65A) Failed to perform this operation. You cannot use the TDMS Advanced Asynchronous I/O functions and the TDMS Advanced Data Reference I/O functions jointly."}, {-68004, "LabVIEW: (Hex 0xFFFEF65C) Failed to manipulate the .tdms file when the file is opened with the TDMS Advanced Open function. You must either use the TDMS Open function to open the .tdms file or use the Advanced TDMS VIs and functions to manipulate the .tdms file."}, {-68003, "LabVIEW: (Hex 0xFFFEF65D) File is opened in asynchronous mode. You must either set the <B>enable asynchronous</B> input of the TDMS Advanced Open function to FALSE or use the TDMS Advanced Asynchronous Write or TDMS Advanced Asynchronous Read function to perform the operation."}, {-68002, "LabVIEW: (Hex 0xFFFEF65E) Failed to reserve file size. If you are running the TDMS Reserve File Size function on Windows with User Account Control enabled, you must run LabVIEW or the application with administrator privileges."}, {-68001, "LabVIEW: (Hex 0xFFFEF65F) Failed to perform the operation. You must use the TDMS Advanced Open function to open the .tdms file."}, {-68000, "LabVIEW: (Hex 0xFFFEF660) Concurrent references to the same .tdms file cannot be opened with different values for the <B>disable buffering?</B> or <B>enable asynchronous?</B> input of the TDMS Advanced Open function."}, {-67750, "LabVIEW: (Hex 0xFFFEF75A) LabVIEW Web Services: Memory Allocation failed."}, {-67508, "LabVIEW: (Hex 0xFFFEF84C) LabVIEW Web Services: An error occurred when extracting the deployed Web service. The file path might be too long. Reduce the length of VI filenames, directory names, or the Web service itself."}, {-67507, "LabVIEW: (Hex 0xFFFEF84D) LabVIEW Web Services: An error occurred when extracting the deployed Web service. Rebuild the Web service by selecting the \"Use LabVIEW 8.x file layout\" option in the Advanced tab of the web Service properties dialog."}, {-67506, "LabVIEW: (Hex 0xFFFEF84E) LabVIEW Web Services: An operating system exception encountered."}, {-67505, "LabVIEW: (Hex 0xFFFEF84F) LabVIEW Web Services: Message received is invalid for the current state of the File Receiver."}, {-67504, "LabVIEW: (Hex 0xFFFEF850) LabVIEW Web Services: Error creating a temporary file."}, {-67503, "LabVIEW: (Hex 0xFFFEF851) LabVIEW Web Services: Invalid message received."}, {-67502, "LabVIEW: (Hex 0xFFFEF852) LabVIEW Web Services: Copying data to or from a LabVIEW terminal failed."}, {-67501, "LabVIEW: (Hex 0xFFFEF853) LabVIEW Web Services: Parse failed."}, {-67500, "LabVIEW: (Hex 0xFFFEF854) LabVIEW Web Services: Memory allocation failed."}, {-67404, "LabVIEW: (Hex 0xFFFEF8B4) LabVIEW Web Services: Web service deployment failed."}, {-67403, "LabVIEW: (Hex 0xFFFEF8B5) LabVIEW Web Services: Unexpected response from the server."}, {-67402, "LabVIEW: (Hex 0xFFFEF8B6) LabVIEW Web Services: Authentication failed."}, {-67401, "LabVIEW: (Hex 0xFFFEF8B7) LabVIEW Web Services: Unable to detect Application Web Server port."}, {-67400, "LabVIEW: (Hex 0xFFFEF8B8) LabVIEW Web Services: Failed to start the Application Web Server."}, {-67306, "LabVIEW: (Hex 0xFFFEF916) LabVIEW Web Services: Invalid session ID specified."}, {-67305, "LabVIEW: (Hex 0xFFFEF917) LabVIEW Web Services: Function not available for service VIs configured for headerless mode."}, {-67304, "LabVIEW: (Hex 0xFFFEF918) LabVIEW Web Services: Function not available for service VIs configured for output terminal mode."}, {-67303, "LabVIEW: (Hex 0xFFFEF919) LabVIEW Web Services: Variable not defined for current session."}, {-67302, "LabVIEW: (Hex 0xFFFEF91A) LabVIEW Web Services: Input Request ID has no associated session."}, {-67301, "LabVIEW: (Hex 0xFFFEF91B) LabVIEW Web Services: Invalid Request ID."}, {-67300, "LabVIEW: (Hex 0xFFFEF91C) LabVIEW Web Services: Internal error in LabVIEW Web services runtime."}, {-67164, "LabVIEW: (Hex 0xFFFEF9A4) LabVIEW Web Services: A non-printable ASCII character was encountered."}, {-67163, "LabVIEW: (Hex 0xFFFEF9A5) LabVIEW Web Services: Error encountered while writing data to the socket."}, {-67162, "LabVIEW: (Hex 0xFFFEF9A6) LabVIEW Web Services: LabVIEW string conversion error."}, {-67161, "LabVIEW: (Hex 0xFFFEF9A7) LabVIEW Web Services: LabVIEW C Interface memory management error."}, {-67160, "LabVIEW: (Hex 0xFFFEF9A8) LabVIEW Web Services: LabVIEW C Interface table not found."}, {-67159, "LabVIEW: (Hex 0xFFFEF9A9) LabVIEW Web Services: LabVIEW application not found."}, {-67158, "LabVIEW: (Hex 0xFFFEF9AA) LabVIEW Web Services: Error encountered while writing session variable."}, {-67157, "LabVIEW: (Hex 0xFFFEF9AB) LabVIEW Web Services: Error encountered while flushing data into the socket."}, {-67156, "LabVIEW: (Hex 0xFFFEF9AC) LabVIEW Web Services: Unknown map error."}, {-67155, "LabVIEW: (Hex 0xFFFEF9AD) LabVIEW Web Services: Request variables associated with the current request not found."}, {-67154, "LabVIEW: (Hex 0xFFFEF9AE) LabVIEW Web Services: Invalid LabVIEW array handle encountered."}, {-67153, "LabVIEW: (Hex 0xFFFEF9AF) LabVIEW Web Services: Session variables defined for the current session not found."}, {-67152, "LabVIEW: (Hex 0xFFFEF9B0) LabVIEW Web Services: The current request not found."}, {-67151, "LabVIEW: (Hex 0xFFFEF9B1) LabVIEW Web Services: Web service active request map not found."}, {-67150, "LabVIEW: (Hex 0xFFFEF9B2) LabVIEW Web Services: Web Service session manager not found."}, {-67043, "LabVIEW: (Hex 0xFFFEFA1D) LabVIEW Web Services: The Web service is currently unavailable because it is still loading, has crashed, or is disabled. Try accessing the service again later or restarting the Web server."}, {-67041, "LabVIEW: (Hex 0xFFFEFA1F) LabVIEW Web Services: Invalid value for input parameter."}, {-67040, "LabVIEW: (Hex 0xFFFEFA20) LabVIEW Web Services: An invalid HTTP method was encountered."}, {-67039, "LabVIEW: (Hex 0xFFFEFA21) LabVIEW Web Services: Invalid character encountered in terminal name."}, {-67038, "LabVIEW: (Hex 0xFFFEFA22) LabVIEW Web Services: Duplicate terminal name encountered."}, {-67037, "LabVIEW: (Hex 0xFFFEFA23) LabVIEW Web Services: An invalid content header was encountered."}, {-67036, "LabVIEW: (Hex 0xFFFEFA24) LabVIEW Web Services: The uploaded file size is too large."}, {-67035, "LabVIEW: (Hex 0xFFFEFA25) LabVIEW Web Services: ESP Error."}, {-67034, "LabVIEW: (Hex 0xFFFEFA26) LabVIEW Web Services: Object not found in the object map."}, {-67033, "LabVIEW: (Hex 0xFFFEFA27) LabVIEW Web Services: A Web service already exists with the input name."}, {-67032, "LabVIEW: (Hex 0xFFFEFA28) LabVIEW Web Services: This type of Web service is not supported."}, {-67031, "LabVIEW: (Hex 0xFFFEFA29) LabVIEW Web Services: Target OS for this Web service differs from the Web server configuration."}, {-67030, "LabVIEW: (Hex 0xFFFEFA2A) LabVIEW Web Services: Unable to load shared library."}, {-67029, "LabVIEW: (Hex 0xFFFEFA2B) LabVIEW Web Services: SetSysAdminMgr function not found in shared library published as a Web service."}, {-67028, "LabVIEW: (Hex 0xFFFEFA2C) LabVIEW Web Services: Finalize method not found in Web services shared library."}, {-67027, "LabVIEW: (Hex 0xFFFEFA2D) LabVIEW Web Services: Resume method not found in Web services shared library."}, {-67026, "LabVIEW: (Hex 0xFFFEFA2E) LabVIEW Web Services: Pause method not found in Web services shared library."}, {-67025, "LabVIEW: (Hex 0xFFFEFA2F) LabVIEW Web Services: Init not found in Web services shared library."}, {-67024, "LabVIEW: (Hex 0xFFFEFA30) LabVIEW Web Services: Run not found in Web services shared library."}, {-67023, "LabVIEW: (Hex 0xFFFEFA31) LabVIEW Web Services: An operating system exception encountered."}, {-67022, "LabVIEW: (Hex 0xFFFEFA32) LabVIEW Web Services: The current service command is not defined for the variable type encountered."}, {-67021, "LabVIEW: (Hex 0xFFFEFA33) LabVIEW Web Services: Error while creating directory."}, {-67020, "LabVIEW: (Hex 0xFFFEFA34) LabVIEW Web Services: Invalid service directory name encountered."}, {-67019, "LabVIEW: (Hex 0xFFFEFA35) LabVIEW Web Services: VI checksum mismatch."}, {-67018, "LabVIEW: (Hex 0xFFFEFA36) LabVIEW Web Services: Shared Variable engine failure."}, {-67017, "LabVIEW: (Hex 0xFFFEFA37) LabVIEW Web Services: No INI file found in service directory."}, {-67016, "LabVIEW: (Hex 0xFFFEFA38) LabVIEW Web Services: File I/O error."}, {-67015, "LabVIEW: (Hex 0xFFFEFA39) LabVIEW Web Services: System is currently in an invalid state for the current message."}, {-67014, "LabVIEW: (Hex 0xFFFEFA3A) LabVIEW Web Services: Invalid message received."}, {-67013, "LabVIEW: (Hex 0xFFFEFA3B) LabVIEW Web Services: More than one INI file encountered in a service directory."}, {-67012, "LabVIEW: (Hex 0xFFFEFA3C) LabVIEW Web Services: Error encountered while parsing INI file."}, {-67011, "LabVIEW: (Hex 0xFFFEFA3D) LabVIEW Web Services: Copying data to the VI terminal(s) failed."}, {-67010, "LabVIEW: (Hex 0xFFFEFA3E) LabVIEW Web Services: An unsupported LabVIEW data type encountered."}, {-67009, "LabVIEW: (Hex 0xFFFEFA3F) LabVIEW Web Services: Call to run a VI failed."}, {-67008, "LabVIEW: (Hex 0xFFFEFA40) LabVIEW Web Services: The VI has not been cached."}, {-67007, "LabVIEW: (Hex 0xFFFEFA41) LabVIEW Web Services: The service has already been registered."}, {-67006, "LabVIEW: (Hex 0xFFFEFA42) LabVIEW Web Services: The VI has already been cached."}, {-67005, "LabVIEW: (Hex 0xFFFEFA43) LabVIEW Web Services: Unknown VI name. Unable to locate the named VI."}, {-67004, "LabVIEW: (Hex 0xFFFEFA44) LabVIEW Web Services: Memory allocation failure."}, {-67003, "LabVIEW: (Hex 0xFFFEFA45) LabVIEW Web Services: Call to create a VI reference failed. The target might not support SSE2 optimization. Disable SSE2 optimization on the <b>Advanced</b> page of the <b>Web Service Properties</b> dialog box before proceeding."}, {-67002, "LabVIEW: (Hex 0xFFFEFA46) LabVIEW Web Services: Call to create a reference to the LabVIEW application failed."}, {-67001, "LabVIEW: (Hex 0xFFFEFA47) LabVIEW Web Services: The Web service is undefined."}, {-67000, "LabVIEW: (Hex 0xFFFEFA48) LabVIEW Web Services: A LabVIEW internal error occurred."}, {-66504, "LabVIEW: (Hex 0xFFFEFC38) The LabVIEW callback VI could not be registered or removed."}, {-66503, "LabVIEW: (Hex 0xFFFEFC39) The Variable run-time engine is not initialized. Ensure that the NI Scan Engine is installed and then restart the target."}, {-66502, "LabVIEW: (Hex 0xFFFEFC3A) Did not find the specified I/O module. Ensure that the specified module name matches the name of the I/O module currently deployed from the project."}, {-66501, "LabVIEW: (Hex 0xFFFEFC3B) I/O module type mismatch. You attempted to read from an output module or write to an input I/O module."}, {-66500, "LabVIEW: (Hex 0xFFFEFC3C) The size of the data array does not match the number of channels in the I/O module."}, {-66491, "LabVIEW: (Hex 0xFFFEFC45) The wait for an I/O scan completion failed due to either a timeout or because the controller shut down."}, {-66490, "LabVIEW: (Hex 0xFFFEFC46) An internal error occurred. The controller was unable to notify user code that the I/O scan completed."}, {-66480, "LabVIEW: (Hex 0xFFFEFC50) A user fault has occurred."}, {-66462, "LabVIEW: (Hex 0xFFFEFC62) The I/O data is not available because the scan engine is not currently running.  Either the scan engine failed to start or stopped because the scan rate was too fast for your installed I/O."}, {-66461, "LabVIEW: (Hex 0xFFFEFC63) The I/O scan was repeatedly late and the NI Scan Engine terminated to ensure controller stability.  Correct the source of lateness and clear all major faults to restart the scan engine."}, {-66460, "LabVIEW: (Hex 0xFFFEFC64) The I/O scan time exceeded the NI Scan Engine period you specified on the Scan Engine page of the target properties dialog box."}, {-66459, "LabVIEW: (Hex 0xFFFEFC65) The configuration for the I/O channel you accessed is not internally consistent due to a pending configuration change. Try to access the channel again after the configuration operation is complete."}, {-66457, "LabVIEW: (Hex 0xFFFEFC67) The I/O Reference has changed."}, {-66456, "LabVIEW: (Hex 0xFFFEFC68) The NI Scan Engine encountered an error while attempting to synchronize with the LabVIEW timing engine."}, {-66455, "LabVIEW: (Hex 0xFFFEFC69) The I/O device must be added to the project and deployed before the NI Scan Engine can use it."}, {-66454, "LabVIEW: (Hex 0xFFFEFC6A) The NI Scan Engine received a request for an I/O driver that is not currently installed on the controller."}, {-66453, "LabVIEW: (Hex 0xFFFEFC6B) The controller experienced an unrecoverable fault that cannot be cleared.  Reboot your controller and contact National Instruments technical support."}, {-66452, "LabVIEW: (Hex 0xFFFEFC6C) Internal error: A component calling the NI Scan Engine failed to comply with the specified interface."}, {-66451, "LabVIEW: (Hex 0xFFFEFC6D) The specified period for the NI Scan Engine is too short for this platform."}, {-66450, "LabVIEW: (Hex 0xFFFEFC6E) The NI Scan Engine cannot perform the requested operation while in Fault mode.  Clear all major faults and try again."}, {-66442, "LabVIEW: (Hex 0xFFFEFC76) The controller encountered an error and was unable to complete the operation."}, {-66432, "LabVIEW: (Hex 0xFFFEFC80) The NI Scan Engine failed to initialize on time, but may function normally given sufficient time.  If the scanned I/O in your application is not updating properly, contact National Instruments technical support."}, {-66431, "LabVIEW: (Hex 0xFFFEFC81) An internal error terminated the NI Scan Engine.  This is an unrecoverable fault."}, {-66430, "LabVIEW: (Hex 0xFFFEFC82) An internal error prevented a scan engine mode transition.  This is an unrecoverable fault."}, {-66420, "LabVIEW: (Hex 0xFFFEFC8C) A fault could not be added because it would exceed the maximum number of faults for the controller."}, {-66411, "LabVIEW: (Hex 0xFFFEFC95) The variable references I/O that has been taken offline by the user.  The value returned is invalid."}, {-66402, "LabVIEW: (Hex 0xFFFEFC9E) The controller did not have enough memory to complete the operation."}, {-66400, "LabVIEW: (Hex 0xFFFEFCA0) A scan engine operation failed because the NI Scan Engine was not yet started.  Ensure that the VI is running on a controller with the NI Scan Engine installed."}, {-66311, "LabVIEW: (Hex 0xFFFEFCF9) An unknown error occurred when using the Programmatic API."}, {-66310, "LabVIEW: (Hex 0xFFFEFCFA) The given buffer is bad."}, {-66309, "LabVIEW: (Hex 0xFFFEFCFB) This error code is not used anywhere yet"}, {-66308, "LabVIEW: (Hex 0xFFFEFCFC) This error code is not used anywhere yet"}, {-66307, "LabVIEW: (Hex 0xFFFEFCFD) This error code is not used anywhere yet"}, {-66306, "LabVIEW: (Hex 0xFFFEFCFE) The input is bad."}, {-66305, "LabVIEW: (Hex 0xFFFEFCFF) There is an error with the deployment process."}, {-66304, "LabVIEW: (Hex 0xFFFEFD00) The given resource is bad."}, {-66303, "LabVIEW: (Hex 0xFFFEFD01) The assembly package is bad."}, {-66301, "LabVIEW: (Hex 0xFFFEFD03) The transaction ID is invalid."}, {-66231, "LabVIEW: (Hex 0xFFFEFD49) An error occurred while trying to revert a change due to a deployment error. Some variables may have an incorrect configuration."}, {-66230, "LabVIEW: (Hex 0xFFFEFD4A) You must use NI-PSP to read or write the value of this I/O Variable. To access the value of this I/O Variable, use a URL with a prefix of ni.var.psp instead of ni.var.io."}, {-66229, "LabVIEW: (Hex 0xFFFEFD4B) The number of elements written to the I/O variable container does not match the number of I/O variables in the container."}, {-66228, "LabVIEW: (Hex 0xFFFEFD4C) Invalid session."}, {-66227, "LabVIEW: (Hex 0xFFFEFD4D) Invalid entry in configuration file."}, {-66226, "LabVIEW: (Hex 0xFFFEFD4E) Incorrect use of internal API for I/O variable."}, {-66225, "LabVIEW: (Hex 0xFFFEFD4F) You cannot write to this I/O alias because it is configured as read only."}, {-66224, "LabVIEW: (Hex 0xFFFEFD50) You cannot read from this I/O alias because it is configured as write-only."}, {-66223, "LabVIEW: (Hex 0xFFFEFD51) The target ran out of memory while trying to configure network publishing of an I/O variable. This variable is no longer published correctly. You can either free some memory and deploy the variable again or restart your system."}, {-66221, "LabVIEW: (Hex 0xFFFEFD53) You cannot scale values of this data type."}, {-66219, "LabVIEW: (Hex 0xFFFEFD55) Network publishing of I/O variables was late."}, {-66218, "LabVIEW: (Hex 0xFFFEFD56) An unexpected error occurred while updating a network-published value."}, {-66217, "LabVIEW: (Hex 0xFFFEFD57) The I/O variable configuration is corrupt and cannot be read."}, {-66216, "LabVIEW: (Hex 0xFFFEFD58) LabVIEW detected a feedback cycle while resolving aliases."}, {-66215, "LabVIEW: (Hex 0xFFFEFD59) The NI Scan Engine has not been initialized or has been shut down."}, {-66214, "LabVIEW: (Hex 0xFFFEFD5A) The alias variable was unable to resolve the parent variable."}, {-66213, "LabVIEW: (Hex 0xFFFEFD5B) Could not deploy variable because a variable of the same name already exists."}, {-66212, "LabVIEW: (Hex 0xFFFEFD5C) The data type of the reference does not match the data type of the variable."}, {-66211, "LabVIEW: (Hex 0xFFFEFD5D) Insufficient memory on target."}, {-66210, "LabVIEW: (Hex 0xFFFEFD5E) Failed to deploy Shared Variable library containing I/O aliases.  A Shared Variable library with the same name without I/O aliases is already deployed to the target.  To deploy the Shared Variable library with I/O aliases you must first undeploy the existing library with the same name."}, {-66209, "LabVIEW: (Hex 0xFFFEFD5F) Failed to initialize a deployed variable at system startup."}, {-66208, "LabVIEW: (Hex 0xFFFEFD60) Invalid variable refnum.  Either the variable was deleted after the reference was opened or a valid reference was never opened."}, {-66207, "LabVIEW: (Hex 0xFFFEFD61) You cannot write to an input channel."}, {-66206, "LabVIEW: (Hex 0xFFFEFD62) A required attribute could not be found during deployment of an I/O variable."}, {-66205, "LabVIEW: (Hex 0xFFFEFD63) The variable object was not found."}, {-66204, "LabVIEW: (Hex 0xFFFEFD64) The data type of the I/O variable alias does not match the data type of the I/O variable itself."}, {-66203, "LabVIEW: (Hex 0xFFFEFD65) This I/O variable requires a hardware driver that is not installed on the deployment target."}, {-66202, "LabVIEW: (Hex 0xFFFEFD66) Unable to force the requested channels."}, {-66201, "LabVIEW: (Hex 0xFFFEFD67) The installed version of nilwpce.dll or nilwpce.out is out of date."}, {-66200, "LabVIEW: (Hex 0xFFFEFD68) An unknown error occurred while using a variable."}, {-66040, "LabVIEW: (Hex 0xFFFEFE08) An internal error occurred. An I/O driver attempted an operation that is not supported by this version of the NI Scan Engine."}, {-66030, "LabVIEW: (Hex 0xFFFEFE12) The operation cannot be completed because one of the scanned I/O buses is not in the required I/O mode."}, {-66023, "LabVIEW: (Hex 0xFFFEFE19) The I/O scan rate cannot be changed at this time due to the state of one of the scanned I/O buses. Try again later."}, {-66022, "LabVIEW: (Hex 0xFFFEFE1A) The specified I/O scan rate is within range, but too precise for one of the scanned I/O buses. Round the rate up or down to the supported resolution."}, {-66021, "LabVIEW: (Hex 0xFFFEFE1B) The specified I/O scan rate is too slow for one of the scanned I/O buses."}, {-66020, "LabVIEW: (Hex 0xFFFEFE1C) The specified I/O scan rate is too fast for one of the scanned I/O buses."}, {-66013, "LabVIEW: (Hex 0xFFFEFE23) An internal error occurred: an I/O plug-in operation requested an invalid I/O collection."}, {-66012, "LabVIEW: (Hex 0xFFFEFE24) An internal error occurred: the specified I/O channel is not present in the specified I/O collection."}, {-66011, "LabVIEW: (Hex 0xFFFEFE25) An internal error occurred: the variable's data size is not consistent with the size of the I/O channel."}, {-66010, "LabVIEW: (Hex 0xFFFEFE26) An internal error occurred: the device identity data is not valid for this I/O plug-in."}, {-66009, "LabVIEW: (Hex 0xFFFEFE27) An internal error occurred: this I/O collection was already added to the I/O scan."}, {-66008, "LabVIEW: (Hex 0xFFFEFE28) The variable belongs to a module or I/O collection that is currently disconnected or offline."}, {-66004, "LabVIEW: (Hex 0xFFFEFE2C) An internal error occurred: an invalid argument was passed to an I/O plug-in."}, {-66001, "LabVIEW: (Hex 0xFFFEFE2F) An I/O plug-in ran out of memory."}, {-66000, "LabVIEW: (Hex 0xFFFEFE30) A miscellaneous system error has occurred in an I/O plug-in."}, {-40635, "LabVIEW: (Hex 0xFFFF6145) The network speed you configured does not match the actual network speed.  This can happen if your network adapter is slower than the network speed you specified or if another adapter, hub, or switch has downgraded the actual network speed."}, {-40634, "LabVIEW: (Hex 0xFFFF6146) The node that owns the associated variable cannot use the \"Data Received\" timing source, or the node that owns the associated variable can use only the \"Data Sent\" timing source."}, {-40633, "LabVIEW: (Hex 0xFFFF6147) The requested error cannot be ignored because a full or partial shutdown of the node and/or network has been initiated."}, {-40632, "LabVIEW: (Hex 0xFFFF6148) LabVIEW has detected a valid packet that does not follow NI's deterministic protocol on the network.  LabVIEW will shut down the node/network."}, {-40631, "LabVIEW: (Hex 0xFFFF6149) An already deployed configuration for one or more network nodes does not match the configuration of this node."}, {-40630, "LabVIEW: (Hex 0xFFFF614A) The network transmission violated the requested timing. Refer to the \"Avoid Jitter\" topic and other timing topics in the LabVIEW Help for information on what may have caused the error and how you can avoid it."}, {-40629, "LabVIEW: (Hex 0xFFFF614B) Resource allocation/creation/configuration failed because the existing resource is configured with different parameters. LabVIEW generates this error when you attempt to recreate a particular resource, such as a channel, with, for example, a different buffer size."}, {-40627, "LabVIEW: (Hex 0xFFFF614D) Read failed after three retries because new data was placed into the buffer."}, {-40626, "LabVIEW: (Hex 0xFFFF614E) The clock synchronization algorithm failed because a certain amount of cycle start packets have been missed. The deterministic communication engine must be restarted before 
